vi "Get List Information.vi"(8 "List Selection":string, 9 "DQMH Modules Info":T3, 10 "References Map":map{string, refnum<vi>}(c390), 11 "Tree Map":T4) -> (0 "Documentation":T2, 1 "Clon?":bool, 2 "Vi out":refnum<vi>, 3 "Module type":T1, 4 "VI Connector Pane":picture, 5 "DQMH Lib":refnum<vi>)   [LabVIEW 2020, in "Panter Dashboard.lvlib"]
uses:
  Panter Dashboard.lvlib
  <vilib>/National Instruments/Tree Map/Tree Map Data.ctl
  Module type--enum.ctl
  DQMH Modules Info--cluster.ctl
  Documentation--cluster.ctl
  <vilib>/National Instruments/Tree Map/Tree Map.lvlib
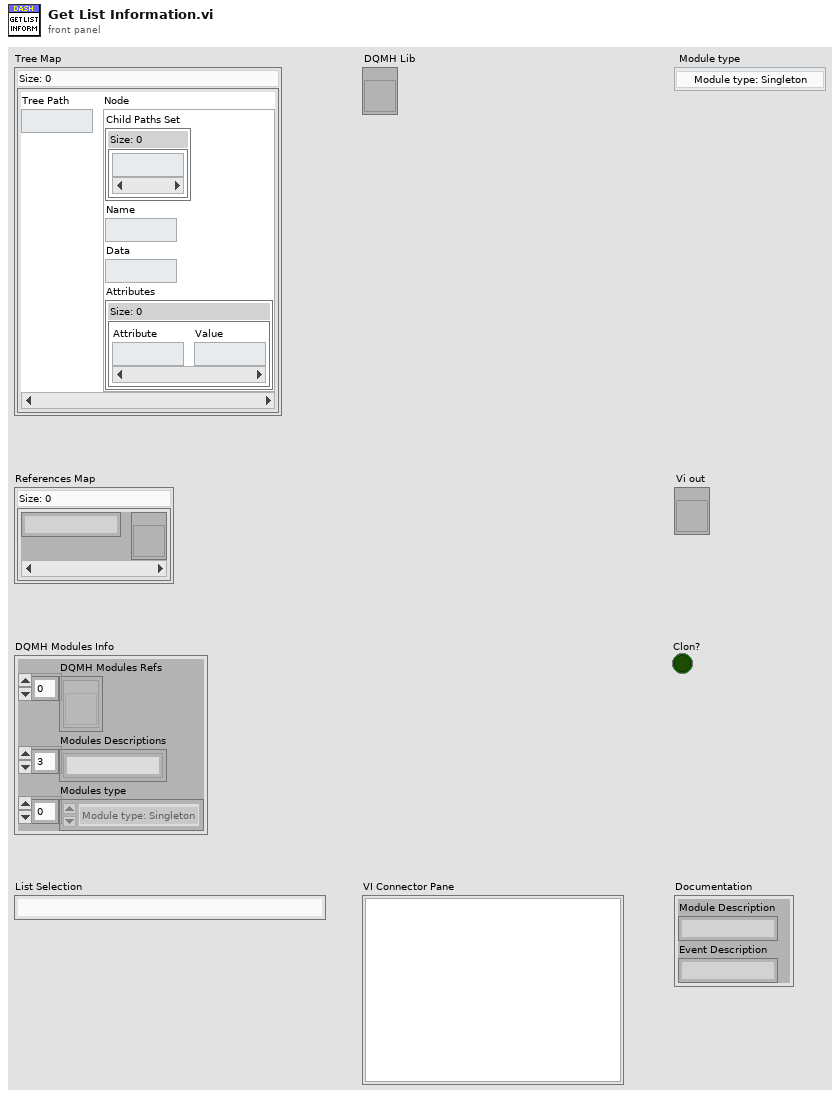
[diagram p1: front panel]
types:
  T1 = typedef "Panter Dashboard.lvlib/Module type--enum.ctl" = enum16{"Module type: Singleton", "Module type: Cloneable"}
  T2 = typedef "Panter Dashboard.lvlib/Documentation--cluster.ctl" = cluster{"Module Description":string, "Event Description":string}
  T3 = typedef "Panter Dashboard.lvlib/DQMH Modules Info--cluster.ctl" = cluster{"DQMH Modules Refs":refnum<vi>[], "Modules Descriptions":string[], "Modules type":T1[]}
  T4 = typedef "Tree Map.lvlib/Tree Map Data.ctl" = map{string, cluster{"Child Paths Set":set{string}, "Name":string, "Data":string, "Attributes":map{string, string}}}
  T5 = cluster{"Child Paths Set":set{string}, "Name":string, "Data":string, "Attributes":map{string, string}}
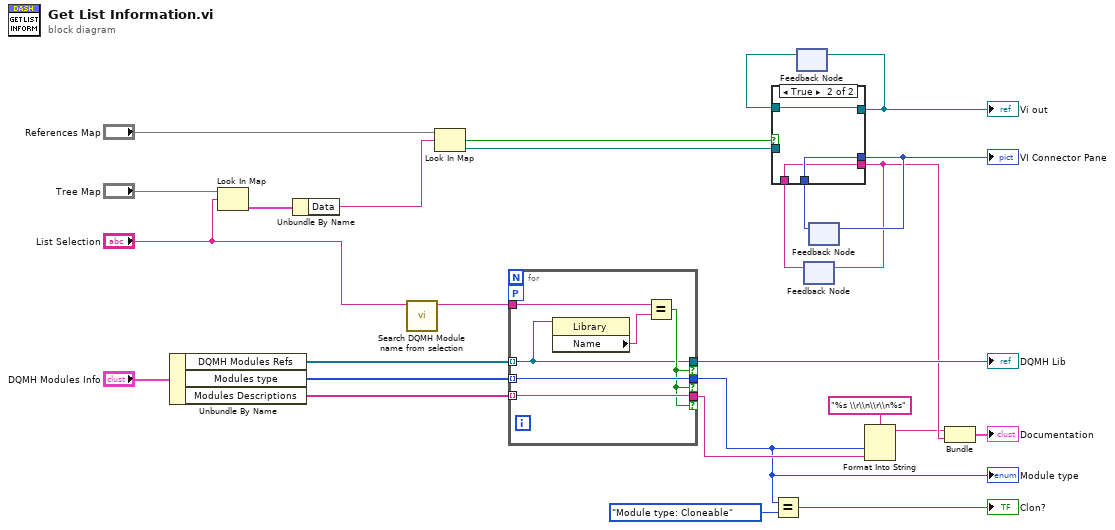
[diagram p0: block diagram]
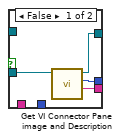
[diagram p2: hidden frame]
diagram:
  n1 = Unbundle By Name("DQMH Modules Info") -> ("DQMH Modules Refs"=w18:refnum<vi>[], "Modules type"=w17:T1[], "Modules Descriptions"=w16:string[])
  n2 = Look In Map(map="Tree Map", key="List Selection") -> (value=w25:T5)  [unwired: 1 in, 1 out]
  n3 = Unbundle By Name(w25) -> ("Data"=w21:string)
  n4 = call "Search DQMH Module name from selection.vi"("Search Module Name"="List Selection") -> ("Module Name"=w15:string)  [unwired: 10 in]
  n5 = Look In Map(map="References Map", key=w21) -> (key not found?=w22:bool, value=w20:refnum<vi>)  [unwired: 1 in]
  n6 = for {
    tunnel: w18 -> [w28] mode=indexing
    tunnel: w17 -> [w31] mode=indexing
    tunnel: w16 -> [w30] mode=indexing
    tunnel: w15 -> [w32]
    tunnel: [w28] -> w13 if=w29
    tunnel: [w31] -> w3 if=w29
    tunnel: [w30] -> w6 if=w29
    workers-P: _ -> [_]
    n7 = property class="Library"(reference=w28) -> ("Name"=w27:string)  [unwired: 1 in, 2 out]
    n8 = Equal?(x=w32, y=w27) -> (x = y?=w29:bool)
  }
  "DQMH Lib" <- w13
  "Module type" <- w3
  n9 = Equal?(x=w3, y=Module_type--enum."Module type: Cloneable") -> (x = y?=→"Clon?":bool)
  n10 = feedback #1() -> (w11:refnum<vi>)  [unwired: 1 in]
  n11 = feedback #2() -> (w7:string)  [unwired: 1 in]
  n12 = feedback #3() -> (w9:picture)  [unwired: 1 in]
  n13 = case shown="True" w22 {
    tunnel: w20 -> [w36 _]
    tunnel: [w35 w38] -> w10
    tunnel: [w34 w39] -> w12
    tunnel: [w33 w37] -> w8
    tunnel: w11 -> [_ w39]
    tunnel: w9 -> [_ w38]
    tunnel: w7 -> [_ w37]
    frame False {
      n14 = call "Get VI Connector Pane image and Description.vi"("VI in"=w36) -> ("VI Description"=w33:string, "VI Connector Pane"=w35:picture, "Vi out"=w34:refnum<vi>)  [unwired: 7 in, 1 out]
    }
    frame True {
    }
  }
  "VI Connector Pane" <- w10
  "Vi out" <- w12
  n15 = feedback-in #1(w12) -> ()
  n16 = feedback-in #2(w8) -> ()
  n17 = feedback-in #3(w10) -> ()
  n18 = Format Into String(format string="%s \\r\\n\\r\\n%s", w3, w6) -> (resulting string=w5:string)  [unwired: 2 in, 1 out]
  n19 = Bundle(w5, "VI Description"=w8) -> (→"Documentation":cluster{string, "VI Description":string})  [unwired: 1 in]
